vi "Register Events.vi"(8 "error in (no error)":errorcluster, 11 "WebView2 Control in":refnum<class "WebView2 Control.lvclass">) -> (0 "error out":errorcluster, 2 "Events":T1, 3 "WebView2 Control out":refnum<class "WebView2 Control.lvclass">)   [LabVIEW 2020, in "WebView2.lvlib" / "WebView2 Control.lvclass"]
uses:
  WebView2 Control.lvclass
  WebView2 Control.lvclass/WebView2 Control.ctl
  _Raise Nav Complete Event.vi
  _Raise Navigation Starting Event.vi
  _Raise Source Changed Event.vi
  _Raise Document Title Changed.vi
  _Raise StatusBarTextChanged.vi
  _Raise WebMessageReceived.vi
  _Raise WindowCloseRequested.vi
  _Raise Dom Content Loaded.vi
  E:/Labview/LV 2020/Libs/WebView2/LV-WebView2/Source/Libs/Microsoft.Web.WebView2.Core.dll
  Libs/Microsoft.Web.WebView2.Core.dll
  Navigation Event Data.ctl
  Source Changed Event Data.ctl
  Navigation Start Event Data.ctl
  Events.ctl
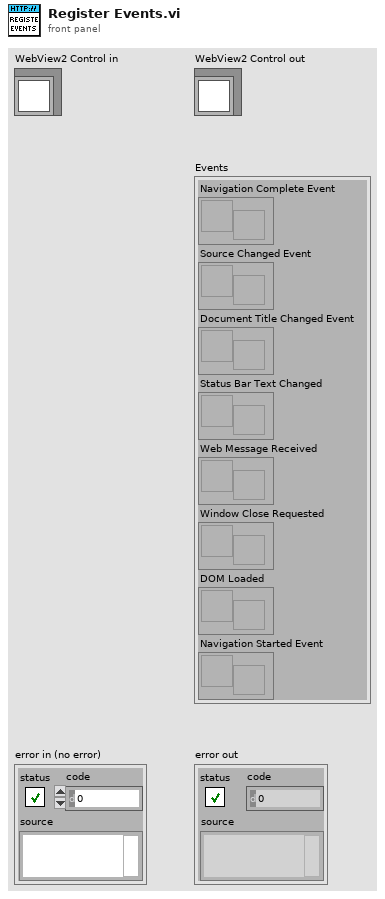
[diagram p1: front panel]
types:
  T1 = typedef "WebView2.lvlib/WebView2 Control.lvclass/Events.ctl" = cluster{"Navigation Complete Event":refnum<user-event>, "Source Changed Event":refnum<user-event>, "Document Title Changed Event":refnum<user-event>, "Status Bar Text Changed":refnum<user-event>, "Web Message Received":refnum<user-event>, "Window Close Requested":refnum<user-event>, "DOM Loaded":refnum<user-event>, "Navigation Started Event":refnum<user-event>}
  T2 = typedef "WebView2.lvlib/WebView2 Control.lvclass/Res.ctl" = cluster{"WebView2":refnum<k24>, "Webview2 Core":refnum<k24>, "event callback":refnum<k27>, "Environment":refnum<k24>}
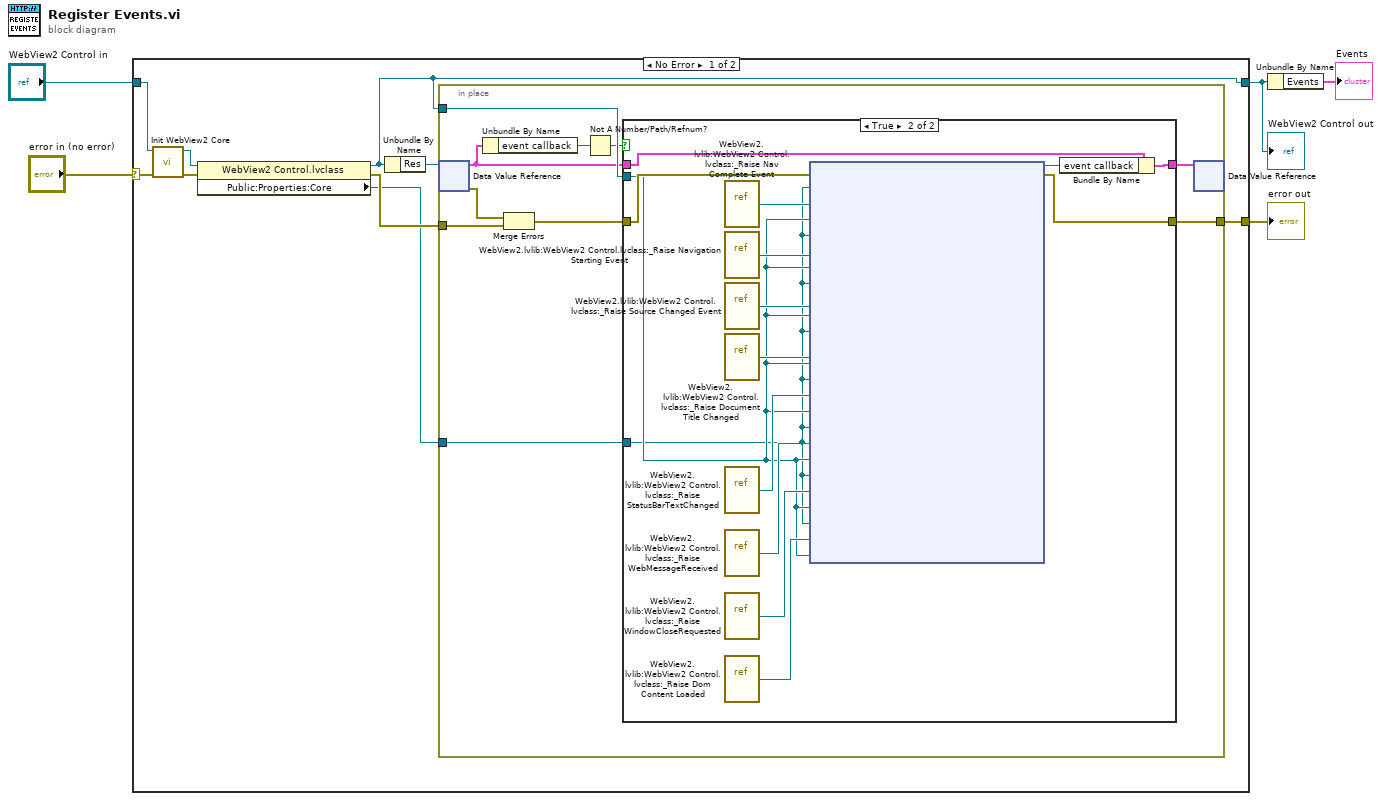
[diagram p0: block diagram]
diagram:
  n1 = case shown="No Error" "error in (no error)" {
    selector: "error in (no error)" -> [w13 w43]
    tunnel: [w7 w42] -> w1
    tunnel: "WebView2 Control in" -> [w14 w42]
    tunnel: [w10 w43] -> w3
    frame No Error {
      n2 = call "Init WebView2 Core.vi"("error in (no error)"=w13, "WebView2"=w14) -> ("error out"=w11:errorcluster, "WebView2.lvlib:WebView2 Control.lvclass"=w8:refnum<class "WebView2 Control.lvclass">)  [unwired: 8 in]
      n3 = property class="WebView2 Control.lvclass"(reference=w8, error in=w11) -> (reference out=w7:refnum<class "WebView2 Control.lvclass">, error out=w9:errorcluster, "Public:Properties:Core"=w6:refnum<k24>)
      n4 = Unbundle By Name(w7) -> ("Res"=w12:refnum<data-value>)
      n5 = in-place {
        in-place-border: w9 -> [w24]
        in-place-border: w7 -> [w21]
        in-place-border: [w20] -> w10
        in-place-border: w6 -> [w15]
        n6 = in-place-dvr #1(w12) -> (w17:T2, w23:errorcluster)
        n7 = Unbundle By Name(w17) -> ("event callback"=w19:refnum<k27>)
        n8 = Merge Errors(w23, w24) -> (w22:errorcluster)
        n9 = Not A Number/Path/Refnum?(number/path/refnum=w19) -> (NaN/Path/Refnum?=w18:bool)
        n10 = case shown="True" w18 {
          tunnel: [w26 w41] -> w20
          tunnel: w22 -> [w26 w37]
          tunnel: w21 -> [_ w28]
          tunnel: w17 -> [w25 w38]
          tunnel: [w25 w39] -> w16
          tunnel: w15 -> [_ w27]
          frame False {
          }
          frame True {
            n11 = vi-ref "WebView2.lvlib:WebView2 Control.lvclass:_Raise Nav Complete Event.vi"() -> (w36:refnum<vi>)
            n12 = vi-ref "WebView2.lvlib:WebView2 Control.lvclass:_Raise Navigation Starting Event.vi"() -> (w35:refnum<vi>)
            n13 = vi-ref "WebView2.lvlib:WebView2 Control.lvclass:_Raise Source Changed Event.vi"() -> (w34:refnum<vi>)
            n14 = vi-ref "WebView2.lvlib:WebView2 Control.lvclass:_Raise Document Title Changed.vi"() -> (w33:refnum<vi>)
            n15 = vi-ref "WebView2.lvlib:WebView2 Control.lvclass:_Raise StatusBarTextChanged.vi"() -> (w32:refnum<vi>)
            n16 = vi-ref "WebView2.lvlib:WebView2 Control.lvclass:_Raise WebMessageReceived.vi"() -> (w31:refnum<vi>)
            n17 = vi-ref "WebView2.lvlib:WebView2 Control.lvclass:_Raise WindowCloseRequested.vi"() -> (w30:refnum<vi>)
            n18 = vi-ref "WebView2.lvlib:WebView2 Control.lvclass:_Raise Dom Content Loaded.vi"() -> (w29:refnum<vi>)
            n19 = node(w37, w27, w36, w28, w27, w35, w28, w27, w34, w28, w27, w33, w28, w27, w32, w28, w27, w31, w28, w27, w30, w28, w27, w29, w28) -> (w40:refnum<k27>, w41:errorcluster)  [unwired: 1 in]
            n20 = Bundle By Name(cluster=w38, "event callback"=w40) -> (w39:T2)
          }
        }
        n21 = in-place-dvr #1(w16) -> ()  [unwired: 2 out]
      }
    }
    frame Error {
    }
  }
  "error out" <- w3
  "WebView2 Control out" <- w1
  n22 = Unbundle By Name(w1) -> ("Events"=→"Events":T1)
